vi "ep_Check dt Constant.vi"(7 "reset? (F)":bool, 8 "error in (no error)":errorcluster, 11 "dt":dbl) -> (0 "error out":errorcluster, 3 "dup dt":dbl)   [LabVIEW 2013, in "NI_EP_Power Measurement.lvlib"]
uses:
  <vilib>/addons/Electrical Power/Power Measurement/NI_EP_Power Measurement.lvlib
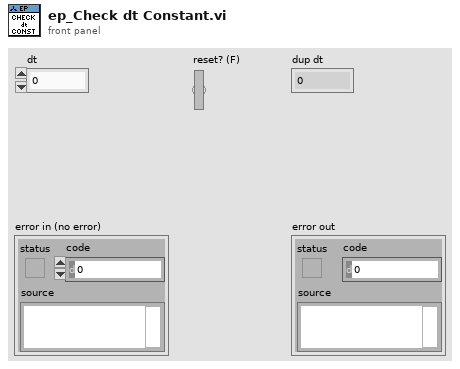
[diagram p1: front panel]
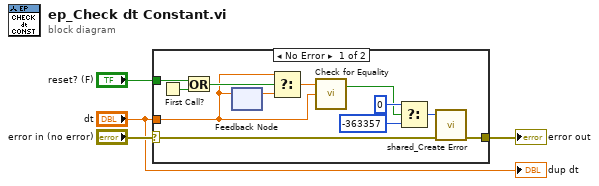
[diagram p0: block diagram]
diagram:
  n1 = case shown="No Error" "error in (no error)" {
    selector: "error in (no error)" -> [w11 w17]
    tunnel: "dt" -> [w6 _]
    tunnel: "reset? (F)" -> [w8 _]
    tunnel: [w13 w17] -> w2
    frame No Error {
      n2 = First Call?() -> (First Call?: T/F=w9:bool)
      n3 = Or(x=w8, y=w9) -> (x .or. y?=w10:bool)
      n4 = feedback-in #1(w6) -> ()
      n5 = feedback #1() -> (w16:dbl)  [unwired: 1 in]
      n6 = Select(t=w6, s=w10, f=w16) -> (s? t:f=w7:dbl)
      n7 = call <vilib>:"Check for Equality.vi"("n2"=w6, "n1"=w7) -> ("equal?"=w5:bool)  [unwired: 2 out]
      n8 = Select(t=0, s=w5, f=-363357) -> (s? t:f=w12:i32)
      n9 = call <vilib>:"shared_Create Error.vi"("error in (no error)"=w11, "error code (0)"=w12) -> ("error out"=w13:errorcluster)  [unwired: 9 in]
    }
    frame Error {
    }
  }
  "error out" <- w2
  "dup dt" <- "dt"
